vi "Add System Mapping.vi"(8 "error in (no error)":errorcluster, 9 "Destinations":string[](array[string]), 10 "Sources":string[](array[string]), 11 "SDF Ref":refnum<k24>) -> (0 "error out":errorcluster)   [LabVIEW 2016, in "System Mapping Tool.lvlib"]
uses:
  System Mapping Tool.lvlib
  NationalInstruments.VeriStand.SystemDefinitionAPI
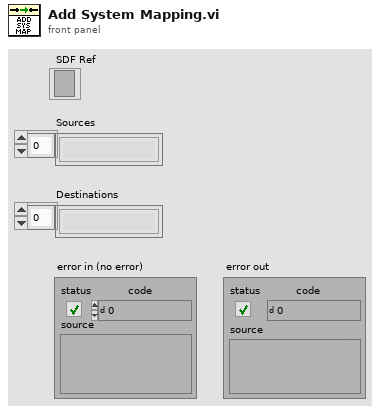
[diagram p1: front panel]
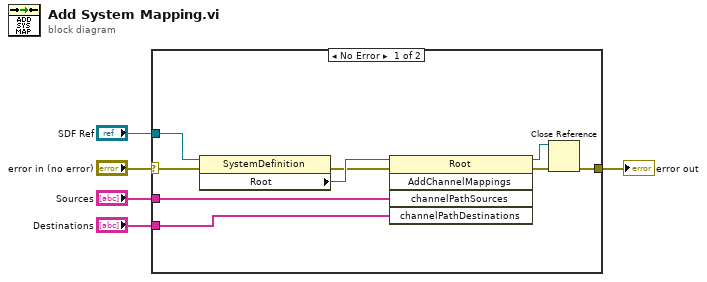
[diagram p0: block diagram]
diagram:
  n1 = case shown="No Error" "error in (no error)" {
    selector: "error in (no error)" -> [w13 w15]
    tunnel: [w10 w15] -> w4
    tunnel: "SDF Ref" -> [w8 _]
    tunnel: "Sources" -> [w7 _]
    tunnel: "Destinations" -> [w6 _]
    frame No Error {
      n2 = property class="SystemDefinition"(reference=w8, error in=w13) -> (error out=w12:errorcluster, "Root"=w14:refnum<k24>)  [unwired: 1 out]
      n3 = invoke class="Root" method="AddChannelMappings"(reference=w14, error in=w12, "channelPathSources"=w7, "channelPathDestinations"=w6) -> (reference out=w9:refnum<k24>, error out=w11:errorcluster)  [unwired: 1 in, 3 out]
      n4 = Close Reference(reference=w9, error in (no error)=w11) -> (error out=w10:errorcluster)
    }
    frame Error {
    }
  }
  "error out" <- w4
